vi "run on executor.vi"(8 "error in":errorcluster, 9 "execution system":T1=enum."standard", 10 "task":refnum<class "task.lvclass">, 11 "dispatcher":refnum<data-value>) -> (0 "error out":errorcluster, 3 "dispatcher out":refnum<data-value>)   [LabVIEW 2013, in "thread pool.lvclass"]
uses:
  thread pool.lvclass
  task/task.lvclass
  execution system.ctl
  task/task.lvclass/task.ctl
  thread pool.lvclass/thread pool.ctl
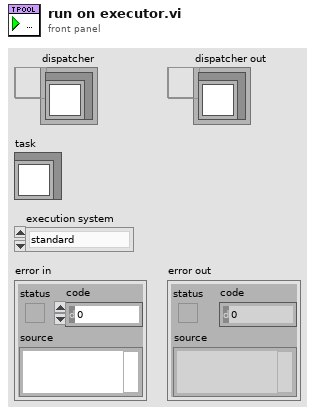
[diagram p1: front panel]
types:
  T1 = typedef "thread pool.lvclass/execution system.ctl" = enum32{"user interface", "standard", "instrument i/o", "data acquisition", "other 1", "other 2"}
  T2 = typedef "thread pool.lvclass/strict executor reference.ctl" = refnum<vi>
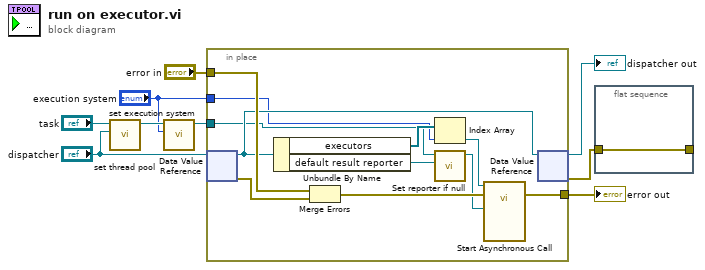
[diagram p0: block diagram]
diagram:
  n1 = call "set thread pool.vi"("dispatcher"="dispatcher", "task in"="task") -> ("task out"=w4:refnum<class "task.lvclass">)  [unwired: 9 in]
  n2 = call "set execution system.vi"("execution system"="execution system", "task in"=w4) -> ("task out"=w2:refnum<class "task.lvclass">)  [unwired: 9 in]
  n3 = in-place {
    in-place-border: "error in" -> [w19]
    in-place-border: [w18] -> w8
    in-place-border: w2 -> [w14]
    in-place-border: "execution system" -> [w10]
    n4 = in-place-dvr #1("dispatcher") -> (w17:refnum<class "thread pool.lvclass">, w15:errorcluster)
    n5 = Unbundle By Name(w17) -> ("executors"=w20:T2[], "default result reporter"=w12:refnum<class "results reporter.lvclass">)
    n6 = Merge Errors(w19, w15) -> (w16:errorcluster)
    n7 = Index Array(array=w20, index=w10) -> (element=w11:T2)
    n8 = call "Set reporter if null.vi"("results reporter"=w12, "task in"=w14) -> ("task out"=w13:refnum<class "task.lvclass">)  [unwired: 9 in]
    n9 = call-by-ref "Start Asynchronous Call"(reference=w11, error in=w16, "task"=w13) -> (error out=w18:errorcluster)  [unwired: 11 in, 1 out]
    n10 = in-place-dvr #1(w17) -> (→"dispatcher out":refnum<data-value>, w6:errorcluster)
  }
  "error out" <- w8
  n11 = flat-sequence {
    tunnel: [w21] -> _
    tunnel: w6 -> [w21]
    frame #0 {
    }
  }
